vi "calculateFrequencyTable.vi"(1 "base-frequency":i32=10000, 2 "frequency-points":i32=18) -> (0 "Array":i32[](array[numeric]))   [LabVIEW 2013]
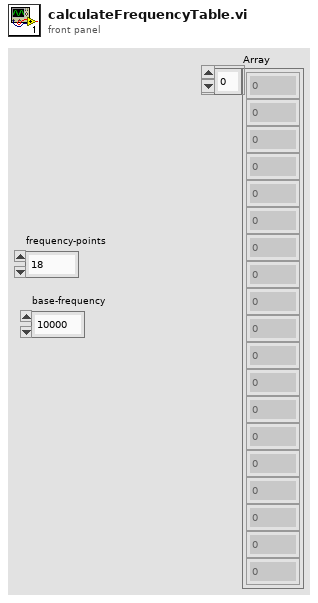
[diagram p1: front panel]
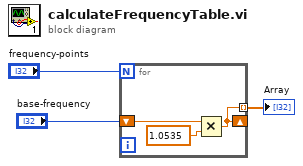
[diagram p0: block diagram]
diagram:
  n1 = for {
    N: "frequency-points" -> [_]
    shift-right: [w4] -> _
    shift-left: "base-frequency" -> [w6]
    tunnel: [w4] -> w1 mode=indexing
    n2 = Multiply(x=w6, y=1.0535) -> (x*y=w4:dbl)
  }
  "Array" <- w1
